vi "Roughness Averager Convex Hull Compute.vi"(8 "error in (no error)":errorcluster, 11 "Roughness Averager in":refnum<class "Roughness Averager.lvclass">) -> (0 "error out":errorcluster, 3 "Roughness Averager out":refnum<class "Roughness Averager.lvclass">)   [LabVIEW 2018, in "Roughness Averager.lvclass"]
uses:
  Roughness Averager.lvclass
  Roughness Averager.lvclass/Roughness Averager.ctl
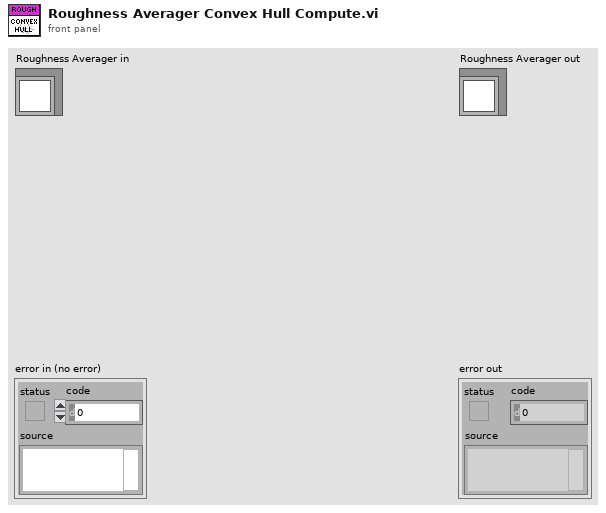
[diagram p1: front panel]
types:
  T1 = typedef "IMAQ Image.ctl" = refnum<image>
  T2 = cluster{"Area":dbl, "Number of Holes":dbl, "Bounding Rect":cluster{"Left":dbl, "Top":dbl, "Right":dbl, "Bottom":dbl}, "Center of Mass":cluster{"X":dbl, "Y":dbl}, "Orientation":dbl, "Dimensions":cluster{"Width":dbl, "Height":dbl}}[]
  T3 = typedef "Video Cam Processor.lvclass/Hull Point STYP.ctl" = cluster{"X":i32, "Y":i32}
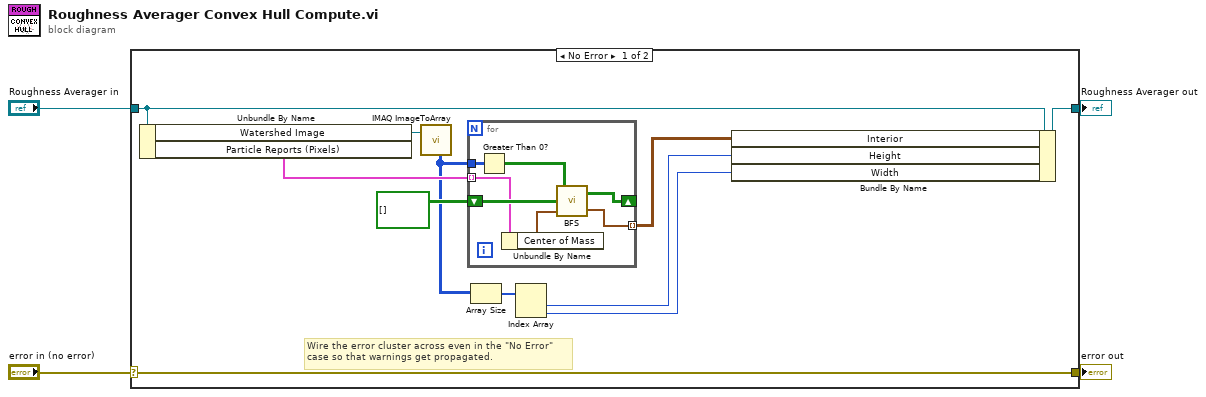
[diagram p0: block diagram]
diagram:
  n1 = case shown="No Error" "error in (no error)" {
    selector: "error in (no error)" -> [w15 w24]
    tunnel: [w15 w24] -> w3
    tunnel: [w5 w23] -> w1
    tunnel: "Roughness Averager in" -> [w11 w23]
    frame No Error {
      # "Wire the error cluster across even in the \"No Error\"\ncase so that warnings get propagated."
      n2 = Unbundle By Name(w11) -> ("Watershed Image"=w14:T1, "Particle Reports (Pixels)"=w13:T2)
      n3 = call "IMAQ ImageToArray"("Image"=w14) -> ("Image Pixels (U16)"=w8:u16[][])  [unwired: 3 in, 4 out]
      n4 = for {
        tunnel: w8 -> [w19]
        tunnel: w13 -> [w17] mode=indexing
        shift-right: [w21] -> _
        shift-left: bool[][] [] -> [w22]
        tunnel: [w20] -> w10 mode=indexing
        n5 = Greater Than 0?(x=w19) -> (x > 0?=w18:bool[][])
        n6 = Unbundle By Name(w17) -> ("Center of Mass"=w16:cluster{"X":dbl, "Y":dbl})
        n7 = call "BFS.vi"("Start (0, 0)"=w16, "Visited"=w22, "Data"=w18) -> ("Valid Coordinates"=w20:T3[], "Visited Out"=w21:bool[][])
      }
      n8 = Array Size(array=w8) -> (size(s)=w9:i32[])
      n9 = Index Array(array=w9) -> (element #1=w7:i32, element #2=w6:i32)  [unwired: 2 in]
      n10 = Bundle By Name(cluster=w11, "Interior"=w10, "Height"=w7, "Width"=w6) -> (w5:refnum<class "Roughness Averager.lvclass">)
    }
    frame Error {
    }
  }
  "error out" <- w3
  "Roughness Averager out" <- w1
